vi "总磷总氮操作日志.vi"(8 "错误输入（无错误）":errorcluster, 11 "data in":T1) -> (0 "错误输出":errorcluster)   [LabVIEW 2016, in "斯坦道总磷.lvlib"]
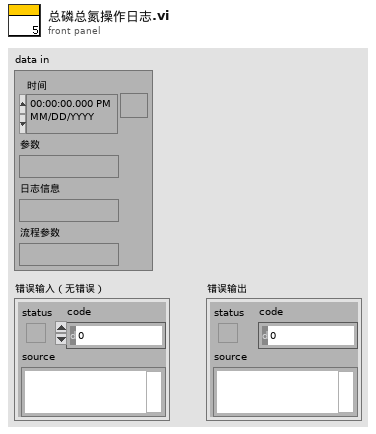
[diagram p1: front panel]
types:
  T1 = typedef "操作日志字段定义.ctl" = cluster{"时间":timestamp, "参数":string, "日志信息":string, "流程参数":string}
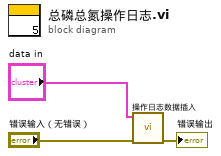
[diagram p0: block diagram]
diagram:
  n1 = call "操作日志数据插入.vi"("data"="data in", "错误输入（无错误）"="错误输入（无错误）") -> ("错误输出"=→"错误输出":errorcluster)  [unwired: 8 in]
